vi "FPGA_target_write_memory.vi"(0 "mem_addr_in":u32, 1 "cmd":u8, 2 "C0":u32, 3 "C1":u32, 4 "data_buffer":u32) -> (14 "mem_addr_out":u32)   [LabVIEW 2014]
doc: "writes data received from the host to an internal memory that will be used later-on"
uses:
  <vilib>/rvi/Emulation/niFpgaSctlEmulationResourceMgr.vi
  <vilib>/rvi/Memory/Memory_Emulation/nirvimemoryEmulationManagerCache_SetValue.vi
  <vilib>/rvi/Emulation/niFpgaSctlEmulationGetInTimedLoop.vi
  <vilib>/rvi/Emulation/niFpgaEmulationIsFPGAContextNoSignature.vi
  <vilib>/rvi/Memory/Memory_Emulation/nirvimemoryEmulationManagerCache_GetValue.vi
  <vilib>/rvi/Memory/Memory_Emulation/nirvimemoryEmulationManagerCache_ReleaseExclusive.vi
  <vilib>/Utility/error.llb/Clear Errors.vi
  <vilib>/rvi/Memory/Memory_Emulation/nirvimemoryEmulationManagerCache_InsertValue.vi
  <vilib>/rvi/Memory/Memory_Emulation/niFpgaMemoryEmulationValidateCache.vi
  <vilib>/rvi/Memory/Memory_Emulation/nirvimemoryEmulationManagerCache_MakeExclusive.vi
  <vilib>/rvi/Memory/Memory_Emulation/niFpgaMemoryEmulationCacheClearOnFirstRun.vi
  <vilib>/rvi/DataTransferAndStorage/Container/Common/niFpgaContainerGetUniqueNameForEmu.vi
  <vilib>/rvi/Memory/Memory_Emulation/nirvimemoryEmulation.vi
  <vilib>/rvi/Memory/Memory_Emulation/nirvimemoryFastEmulation.vi
  <vilib>/rvi/DataTransferAndStorage/Container/XNode/niFpgaContainer.xnode
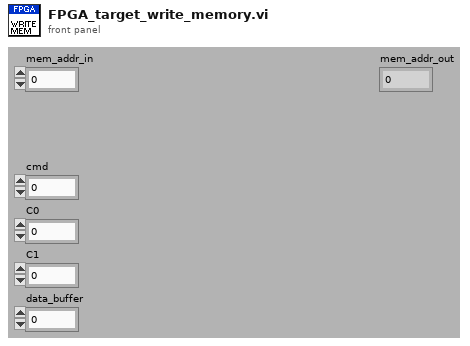
[diagram p1: front panel]
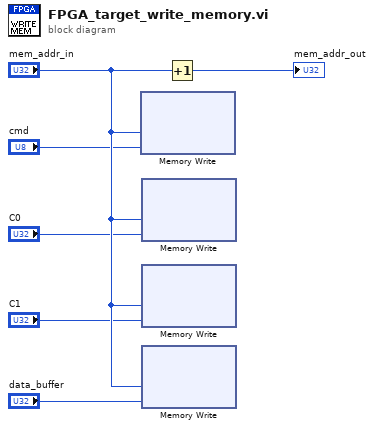
[diagram p0: block diagram]
diagram:
  n1 = xnode ("Memory Write")("Address"="mem_addr_in", "Data"="cmd") -> ()  [unwired: 1 in, 1 out]
  n2 = xnode ("Memory Write")("Address"="mem_addr_in", "Data"="C0") -> ()  [unwired: 1 in, 1 out]
  n3 = xnode ("Memory Write")("Address"="mem_addr_in", "Data"="C1") -> ()  [unwired: 1 in, 1 out]
  n4 = xnode ("Memory Write")("Address"="mem_addr_in", "Data"="data_buffer") -> ()  [unwired: 1 in, 1 out]
  n5 = Increment(x="mem_addr_in") -> (x+1=→"mem_addr_out":u32)
